vi "GlobalBoardIDs.vi"() -> ()   [LabVIEW 2015]
panel:
  in  "Board ID #s":dbl[](array[numeric])
  in  "Board Names":string[](array[string])
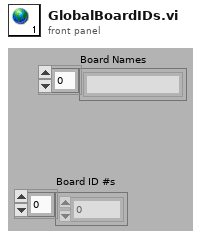
[diagram p1: front panel]
diagram:
